vi "SSC DCPower Filter Sites.vi"(0 "DCPower SSC in":T1[](array[typedef]), 5 "Requested Sites":i32[](array[numeric]), 11 "error in":errorcluster) -> (4 "Filtered DCPower SSC out":T1[](array[typedef]), 15 "error out":errorcluster)   [LabVIEW 2019]
doc: "This VI filters the SSC array to requested sites."
uses:
  SSC DCPower/SSC DCPower.ctl
  Shared SubVIs/Trim Whitespace [Inlined].vi
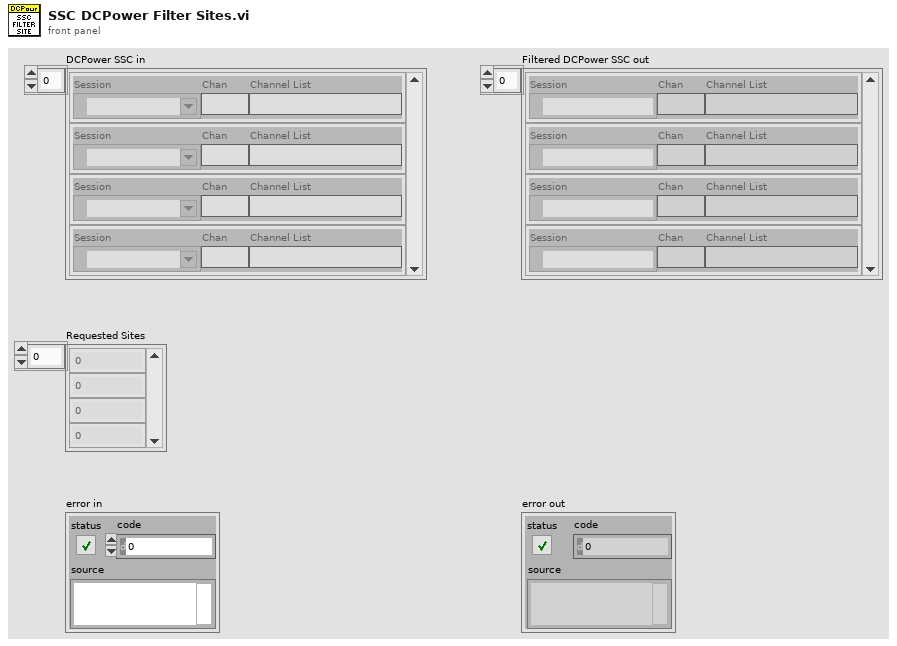
[diagram p1: front panel]
types:
  T1 = typedef "SSC DCPower.ctl" = cluster{"Session":refnum<k15>, "Chan":string, "Channel List":string}
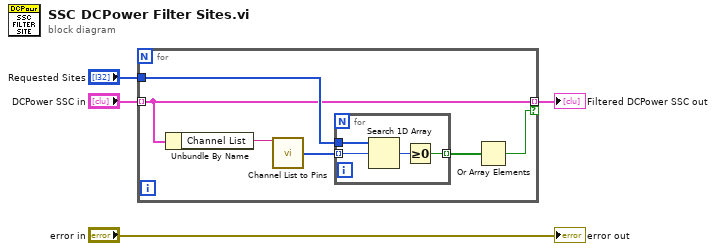
[diagram p0: block diagram]
diagram:
  n1 = for {
    tunnel: "DCPower SSC in" -> [w9] mode=indexing
    tunnel: "Requested Sites" -> [w10]
    tunnel: [w9] -> w1 mode=indexing if=w5
    n2 = Unbundle By Name(w9) -> ("Channel List"=w7:string)
    n3 = call "Channel List to Pins.vi"("Channel List"=w7) -> ("Sites"=w6:i32[])  [unwired: 12 in, 2 out]
    n4 = for {
      tunnel: w10 -> [w14]
      tunnel: [w12] -> w8 mode=indexing
      tunnel: w6 -> [w11] mode=indexing
      n5 = Search 1D Array(1D array=w14, element=w11) -> (index of element=w13:i32)  [unwired: 1 in]
      n6 = Greater Or Equal To 0?(x=w13) -> (x >= 0?=w12:bool)
    }
    n7 = Or Array Elements(Boolean array=w8) -> (logical OR=w5:bool)
  }
  "Filtered DCPower SSC out" <- w1
  "error out" <- "error in"
